vi "Write DigitalInputDevRef.vi"(8 "error in (no error)":errorcluster, 10 "DigitalInputDevRef":T1, 11 "Catapult in":refnum<class "Catapult.lvclass">) -> (0 "error out":errorcluster, 3 "Catapult out":refnum<class "Catapult.lvclass">)   [LabVIEW 2013, in "Catapult.lvclass"]
uses:
  Catapult.lvclass
  <vilib>/Rock Robotics/WPI/DigitalInput/WPI_DigitalInputDevRef.ctl
  <vilib>/Rock Robotics/SystemInterfaces/DIO/FPGA_DIOChannel.ctl
  <vilib>/Rock Robotics/SystemInterfaces/Typedef/FPGA_TypedefDigitalModule.ctl
  Catapult.lvclass/Catapult.ctl
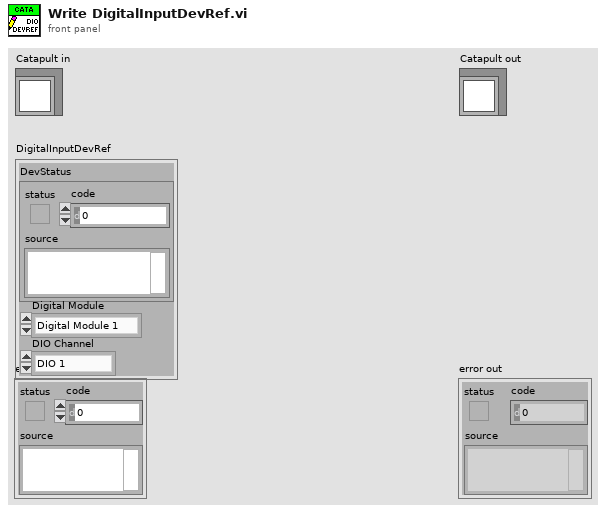
[diagram p1: front panel]
types:
  T1 = typedef "WPI_DigitalInputDevRef.ctl" = cluster{"DevStatus":errorcluster, "DIO Channel":T2, "Digital Module":T3}
  T2 = typedef "FPGA_DIOChannel.ctl" = enum8{"DIO 1", "DIO 2", "DIO 3", "DIO 4", "DIO 5", "DIO 6", "DIO 7", "DIO 8", "DIO 9", "DIO 10", "DIO 11", "DIO 12", "DIO 13", "DIO 14", "Invalid"}
  T3 = typedef "FPGA_TypedefDigitalModule.ctl" = enum16{"Digital Module 1", "Digital Module 2"}
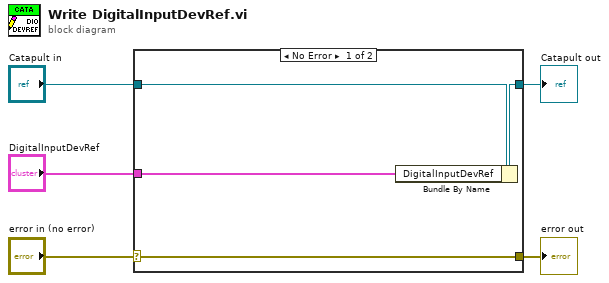
[diagram p0: block diagram]
diagram:
  n1 = case shown="No Error" "error in (no error)" {
    selector: "error in (no error)" -> [w9 w10]
    tunnel: [w9 w10] -> w4
    tunnel: [w7 w11] -> w2
    tunnel: "Catapult in" -> [w8 w11]
    tunnel: "DigitalInputDevRef" -> [w6 _]
    frame No Error {
      n2 = Bundle By Name(cluster=w8, "DigitalInputDevRef"=w6) -> (w7:refnum<class "Catapult.lvclass">)
    }
    frame Error {
    }
  }
  "error out" <- w4
  "Catapult out" <- w2
